vi "op_rel_v6.vi"() -> ()   [LabVIEW 2010]
panel:
  out "Numeric":dbl=240.0
  in  "Knob":u8(knob)=3 scale=0.0..7.0
  out "L0":bool=TRUE
  out "L1":bool=TRUE
  out "L2":bool=TRUE
  out "L3":bool=TRUE
  out "L4":bool
  out "L5":bool
  out "L6":bool
  out "L7":bool
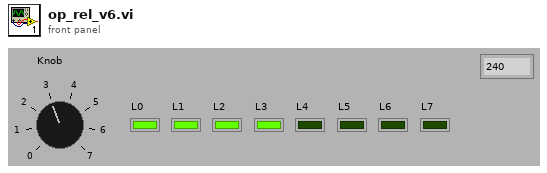
[diagram p1: front panel]
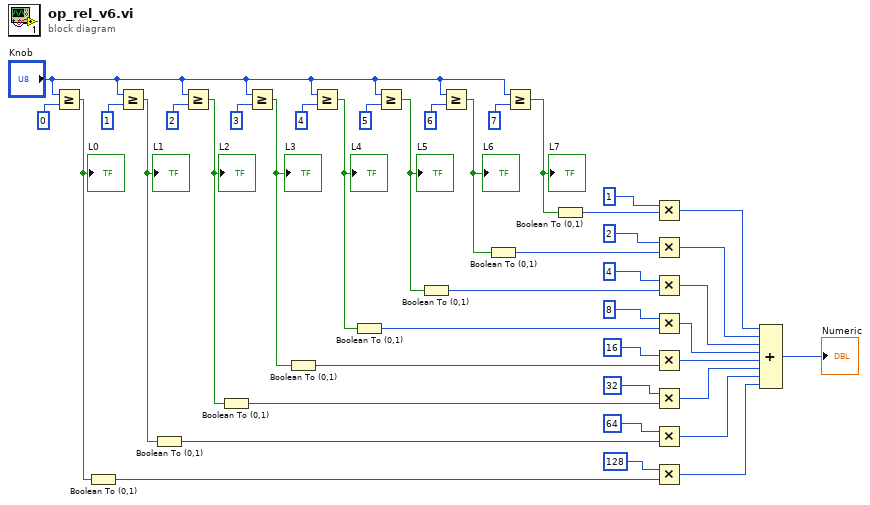
[diagram p0: block diagram]
diagram:
  n1 = Greater Or Equal?(x="Knob", y=0) -> (x >= y?=w16:bool)
  "L0" <- w16
  n2 = Boolean To (0,1)(Boolean=w16) -> (0, 1=w1:i16)
  n3 = Greater Or Equal?(x="Knob", y=1) -> (x >= y?=w8:bool)
  "L1" <- w8
  n4 = Boolean To (0,1)(Boolean=w8) -> (0, 1=w2:i16)
  n5 = Greater Or Equal?(x="Knob", y=2) -> (x >= y?=w9:bool)
  "L2" <- w9
  n6 = Boolean To (0,1)(Boolean=w9) -> (0, 1=w3:i16)
  n7 = Greater Or Equal?(x="Knob", y=3) -> (x >= y?=w10:bool)
  "L3" <- w10
  n8 = Boolean To (0,1)(Boolean=w10) -> (0, 1=w4:i16)
  n9 = Greater Or Equal?(x="Knob", y=4) -> (x >= y?=w11:bool)
  "L4" <- w11
  n10 = Boolean To (0,1)(Boolean=w11) -> (0, 1=w5:i16)
  n11 = Greater Or Equal?(x="Knob", y=5) -> (x >= y?=w7:bool)
  "L5" <- w7
  n12 = Boolean To (0,1)(Boolean=w7) -> (0, 1=w6:i16)
  n13 = Greater Or Equal?(x="Knob", y=6) -> (x >= y?=w13:bool)
  "L6" <- w13
  n14 = Boolean To (0,1)(Boolean=w13) -> (0, 1=w12:i16)
  n15 = Greater Or Equal?(x="Knob", y=7) -> (x >= y?=w15:bool)
  "L7" <- w15
  n16 = Boolean To (0,1)(Boolean=w15) -> (0, 1=w14:i16)
  n17 = Multiply(x=1, y=w14) -> (x*y=w25:i32)
  n18 = Multiply(x=2, y=w12) -> (x*y=w24:i32)
  n19 = Multiply(x=4, y=w6) -> (x*y=w23:i32)
  n20 = Multiply(x=8, y=w5) -> (x*y=w22:i32)
  n21 = Multiply(x=16, y=w4) -> (x*y=w21:i32)
  n22 = Multiply(x=32, y=w3) -> (x*y=w20:i32)
  n23 = Multiply(x=64, y=w2) -> (x*y=w19:i32)
  n24 = Multiply(x=128, y=w1) -> (x*y=w18:i32)
  n25 = Compound Arithmetic op=ADD(w25, w24, w23, w22, w21, w20, w19, w18) -> (→"Numeric":i32)
